vi "界面UI.vi"() -> ()   [LabVIEW 2016]
uses:
  <vilib>/Utility/config.llb/NI_LVConfig.lvlib
panel:
  in  "修改超标留样型号":bool
  out "x=y?":bool
  in  "锁":bool
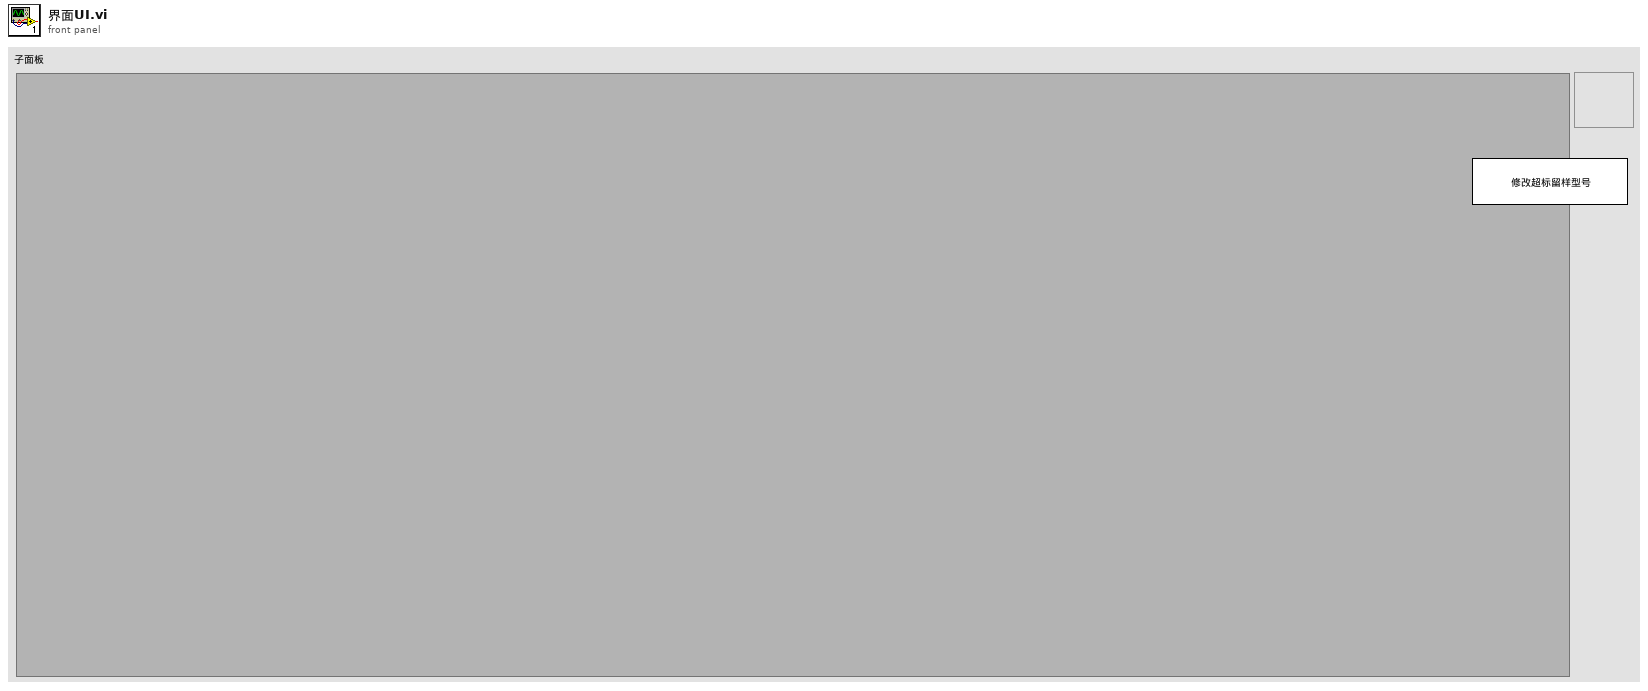
[diagram p1: front panel]
types:
  T1 = typedef "NI_LVConfig.lvlib/Config Data RefNum.ctl" = refnum<k1>
  T2 = enum16{"德润DR803M", "德润DR803L", "德润DR803F", "科盛超标留样"}
  T3 = enum32{"Bad", "Idle", "Run top level", "Running"}
  T4 = cluster{"当前瓶号：":dbl, "平行样：":dbl, "留样瓶数：":dbl, "每瓶次数：":dbl, "每次留样：":dbl, "时间间隔：":dbl, "COD联机：":u16, "氨氮联机：":u16, "4mA浓度：":dbl, "20mA浓度：":dbl, "超标浓度：":dbl, "4mA浓度：":dbl, "20mA浓度:":dbl, "超标浓度：":dbl}
  T5 = cluster{"工作状态":u16, "工作进程":u16, "仪器时间":timestamp, "采样模式":u16, "当前瓶号":dbl, "采样瓶数":dbl, "每瓶采样次数":dbl, "当前瓶已采次数":dbl, "当前瓶采样量":dbl, "采样量定量":dbl, "采样量比例":dbl, "瞬时流量":dbl, "累积流量":dbl, "外置泵状态":dbl, "采样泵状态":dbl, "采样泵方向":dbl, "采样阀":dbl, "采样瓶转盘":dbl, "排水阀":dbl, "清洗泵":dbl, "清洗管工作":dbl, "清洗管电源":dbl, "清洗管运行方向":dbl, "门状态":u16, "采水管有水检测":dbl}
  T6 = cluster{"确定":bool, "单选按钮":enum32{"德润DR803M", "德润DR803L", "德润DR803F", "科盛超标留样"}}
  T7 = enum32{"德润DR803M", "德润DR803L", "德润DR803F", "科盛超标留样"}
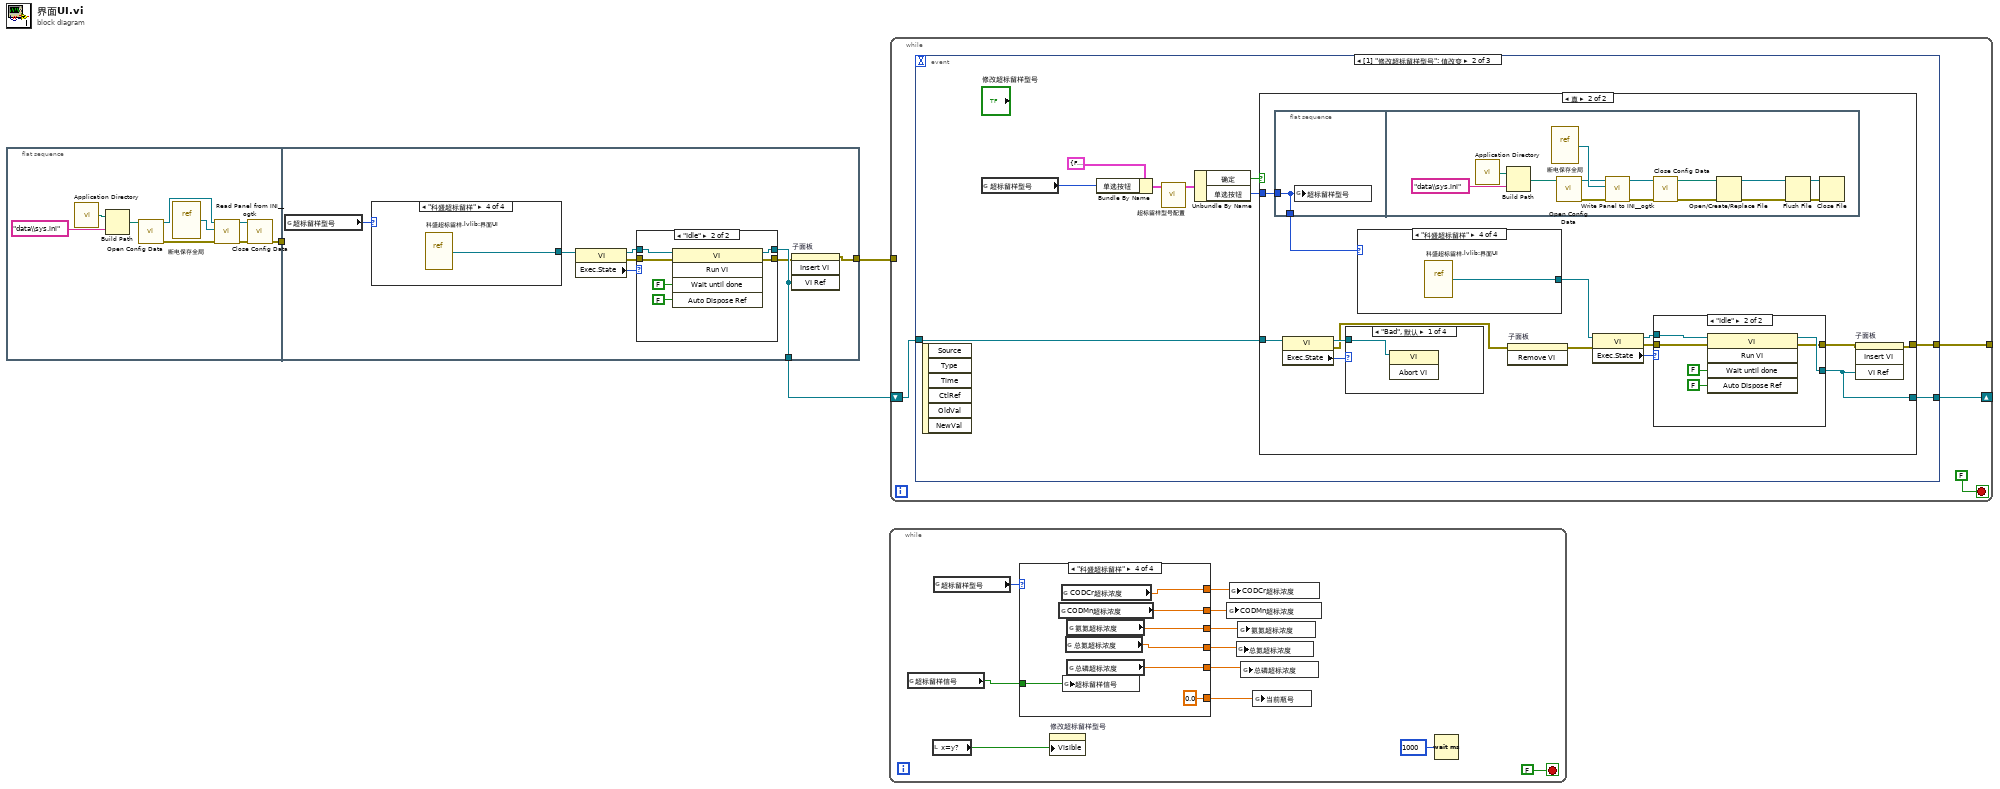
[diagram p0: block diagram]
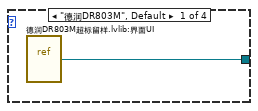
[diagram p2: hidden frame]
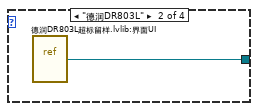
[diagram p3: hidden frame]
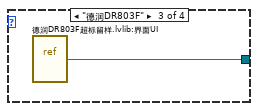
[diagram p4: hidden frame]
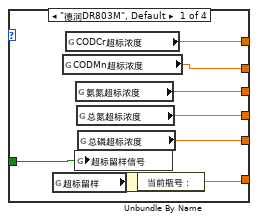
[diagram p6: hidden frame]
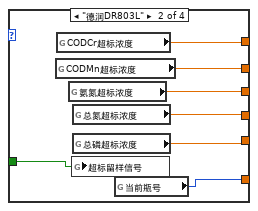
[diagram p7: hidden frame]
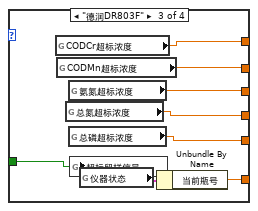
[diagram p8: hidden frame]
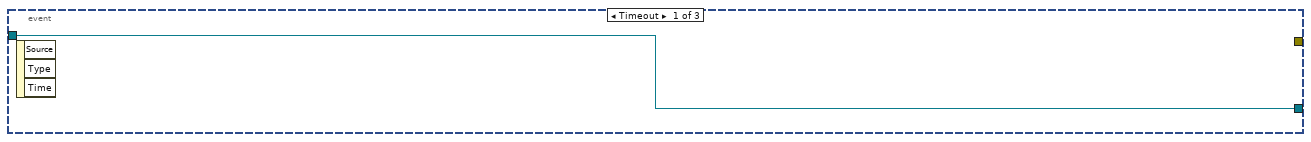
[diagram p9: hidden frame]
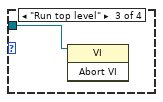
[diagram p12: hidden frame]
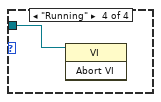
[diagram p13: hidden frame]
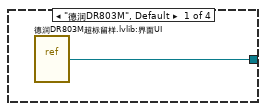
[diagram p14: hidden frame]
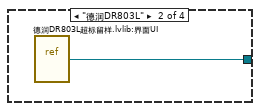
[diagram p15: hidden frame]
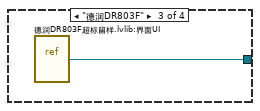
[diagram p16: hidden frame]
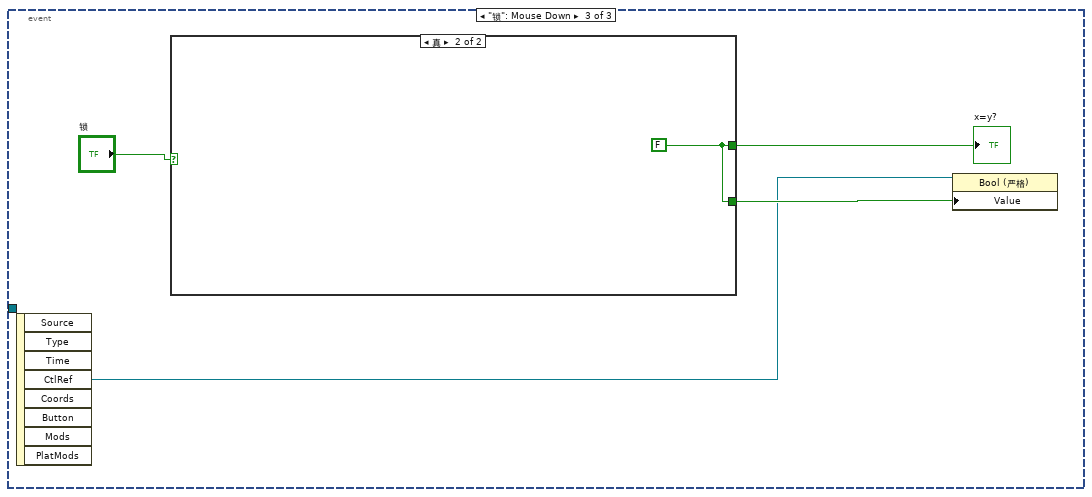
[diagram p18: hidden frame]
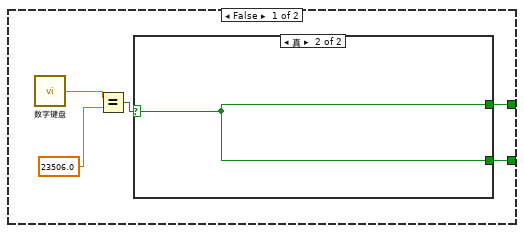
[diagram p19: hidden frame]
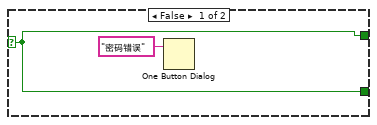
[diagram p20: hidden frame]
diagram:
  n1 = flat-sequence {
    tunnel: [w4] -> w1
    tunnel: [w15] -> w3
    tunnel: [w13] -> w2
    tunnel: w1 -> [_]
    frame #0 {
      n2 = call <vilib>:"Application Directory.vi"() -> ("Application Directory"=w5:path)
      n3 = Build Path(base path=w5, name or relative path="data\\sys.ini" ("名称或相对路径")) -> (appended path=w7:path)
      n4 = call <vilib>:"Open Config Data.vi"("configuration file path"=w7) -> ("error out"=w11:errorcluster, "refnum"=w8:T1)  [unwired: 8 in, 1 out]
      n5 = vi-ref "断电保存全局.vi"() -> (w9:refnum<vi>)
      n6 = call <userlib>:"Read Panel from INI__ogtk.vi"("error in (no error)"=w11, "VI ref"=w9, "refnum"=w8) -> ("error out"=w12:errorcluster, "refnum out"=w10:T1)  [unwired: 7 in]
      n7 = call <vilib>:"Close Config Data.vi"("error in (no error)"=w12, "refnum"=w10) -> ("error out"=w4:errorcluster)  [unwired: 8 in, 1 out]
    }
    frame #1 {
      n8 = global read "断电保存全局.vi" "超标留样型号"() -> (w16:T2)
      n9 = case shown="\"科盛超标留样\"" w16 {
        tunnel: [w21 w22 w23 w24] -> w17
        frame "德润DR803M", Default {
          n10 = vi-ref "德润DR803M超标留样.lvlib:界面UI.vi"() -> (w21:refnum<vi>)
        }
        frame "德润DR803L" {
          n11 = vi-ref "德润DR803L超标留样.lvlib:界面UI.vi"() -> (w22:refnum<vi>)
        }
        frame "德润DR803F" {
          n12 = vi-ref "德润DR803F超标留样.lvlib:界面UI.vi"() -> (w23:refnum<vi>)
        }
        frame "科盛超标留样" {
          n13 = vi-ref "科盛超标留样.lvlib:界面UI.vi"() -> (w24:refnum<vi>)
        }
      }
      n14 = property class="VI"(reference=w17) -> (reference out=w19:refnum<vi>, error out=w18:errorcluster, "Exec.State"=w20:T3)  [unwired: 1 in]
      n15 = case shown="\"Idle\"" w20 {
        tunnel: w19 -> [w26 w32]
        tunnel: [w26 w29] -> w15
        tunnel: w18 -> [w25 w28]
        tunnel: [w25 w27] -> w14
        frame "Bad", Default {
        }
        frame "Idle" {
          n16 = invoke class="VI" method="Run VI"(reference=w32, error in=w28, "Wait until done"=FALSE ("结束前等待"), "Auto Dispose Ref"=FALSE ("自动销毁引用")) -> (reference out=w29:refnum<vi>, error out=w27:errorcluster)  [unwired: 1 in, 3 out]
        }
      }
      n17 = invoke on="子面板" class="SubPnl" method="Insert VI"(error in=w14, "VI Ref"=w15) -> (error out=w13:errorcluster)  [unwired: 2 in, 3 out]
    }
  }
  n18 = while {
    stop <- FALSE stop-if-true
    n19 = global read "外部交互全局.vi" "超标留样信号"() -> (w35:bool)
    n20 = local read "x=y?"() -> (w34:bool)
    n21 = global read "断电保存全局.vi" "超标留样型号"() -> (w41:T2)
    n22 = case shown="\"科盛超标留样\"" w41 {
      tunnel: [w51 w58 w66 w73] -> w40
      tunnel: [w50 w57 w65 w72] -> w39
      tunnel: [w49 w56 w64 w71] -> w38
      tunnel: [w48 w55 w63 w70] -> w37
      tunnel: [w47 w54 w62 w69] -> w36
      tunnel: w35 -> [w46 w53 w61 w68]
      tunnel: [w44 w52 w59 0.0 ("当前瓶号")] -> w33
      frame "德润DR803M", Default {
        n23 = global read "超标留样全局.vi" "超标留样"() -> (w45:T4)
        n24 = global read "超标留样全局.vi" "CODMn超标浓度"() -> (w50:dbl)
        n25 = global read "超标留样全局.vi" "CODCr超标浓度"() -> (w51:dbl)
        n26 = global write "超标留样全局.vi" "超标留样信号"(w46) -> ()
        n27 = global read "超标留样全局.vi" "氨氮超标浓度"() -> (w49:dbl)
        n28 = global read "超标留样全局.vi" "总氮超标浓度"() -> (w48:dbl)
        n29 = global read "超标留样全局.vi" "总磷超标浓度"() -> (w47:dbl)
        n30 = Unbundle By Name(w45) -> ("当前瓶号："=w44:dbl)
      }
      frame "德润DR803L" {
        n31 = global read "串口参数断电保存全局变量.vi" "CODMn超标浓度"() -> (w57:dbl)
        n32 = global read "串口参数断电保存全局变量.vi" "CODCr超标浓度"() -> (w58:dbl)
        n33 = global read "串口参数断电保存全局变量.vi" "氨氮超标浓度"() -> (w56:dbl)
        n34 = global write "串口参数断电保存全局变量.vi" "超标留样信号"(w53) -> ()
        n35 = global read "串口参数断电保存全局变量.vi" "总氮超标浓度"() -> (w55:dbl)
        n36 = global read "串口参数断电保存全局变量.vi" "总磷超标浓度"() -> (w54:dbl)
        n37 = global read "超标留样全局.vi" "当前瓶号"() -> (w52:u16)
      }
      frame "德润DR803F" {
        n38 = global read "超标留样全局.vi" "CODCr超标浓度"() -> (w66:dbl)
        n39 = global read "超标留样全局.vi" "CODMn超标浓度"() -> (w65:dbl)
        n40 = global read "超标留样全局.vi" "总氮超标浓度"() -> (w63:dbl)
        n41 = global read "超标留样全局.vi" "氨氮超标浓度"() -> (w64:dbl)
        n42 = global read "超标留样全局.vi" "总磷超标浓度"() -> (w62:dbl)
        n43 = global write "超标留样全局.vi" "超标留样信号"(w61) -> ()
        n44 = global read "超标留样全局.vi" "仪器状态"() -> (w60:T5)
        n45 = Unbundle By Name(w60) -> ("当前瓶号"=w59:dbl)
      }
      frame "科盛超标留样" {
        n46 = global read "超标留样全局.vi" "CODMn超标浓度"() -> (w72:dbl)
        n47 = global read "超标留样全局.vi" "CODCr超标浓度"() -> (w73:dbl)
        n48 = global write "超标留样全局.vi" "超标留样信号"(w68) -> ()
        n49 = global read "超标留样全局.vi" "总氮超标浓度"() -> (w70:dbl)
        n50 = global read "超标留样全局.vi" "氨氮超标浓度"() -> (w71:dbl)
        n51 = global read "超标留样全局.vi" "总磷超标浓度"() -> (w69:dbl)
      }
    }
    n52 = property on="修改超标留样型号" class="Bool"("Visible"=w34) -> ()  [unwired: 2 in, 2 out]
    n53 = global write "外部交互全局.vi" "CODMn超标浓度"(w39) -> ()
    n54 = global write "外部交互全局.vi" "CODCr超标浓度"(w40) -> ()
    n55 = global write "外部交互全局.vi" "总氮超标浓度"(w37) -> ()
    n56 = global write "外部交互全局.vi" "氨氮超标浓度"(w38) -> ()
    n57 = global write "外部交互全局.vi" "总磷超标浓度"(w36) -> ()
    n58 = global write "外部交互全局.vi" "当前瓶号"(w33) -> ()
    n59 = Wait (ms)(milliseconds to wait=u32 1000 ("等待时间（毫秒）")) -> ()  [unwired: 1 out]
  }
  n60 = while {
    tunnel: [w77] -> _
    tunnel: w2 -> [_]
    shift-right: [w75] -> _
    shift-left: w3 -> [w74]
    stop <- FALSE stop-if-true
    n61 = event shown="[1] \"修改超标留样型号\": 值改变" {
      selector: _ -> [_ _ _]
      dyn-events: _ -> [_ _ _]
      timeout: _ -> [_ _ _]
      tunnel: [_ w81 _] -> w77
      tunnel: [w78 w80 _] -> w75
      tunnel: w74 -> [w78 w79 _]
      event Timeout {
        n62 = event-data() -> ()  [unwired: 1 in, 3 out]
      }
      event "修改超标留样型号": Value Change {
        n63 = event-data() -> ()  [unwired: 1 in, 6 out]
        n64 = global read "断电保存全局.vi" "超标留样型号"() -> (w87:T2)
        n65 = Bundle By Name(cluster=T6 {"确定"=FALSE, "单选按钮"=enum."德润DR803F"} ("输入"), "单选按钮"=w87) -> (w85:T6)
        n66 = call "超标留样型号配置.vi"("输入"=w85) -> ("输出"=w84:T6)  [unwired: 10 in]
        n67 = Unbundle By Name(w84) -> ("确定"=w82:bool, "单选按钮"=w83:T7)
        n68 = case shown="真" w82 {
          tunnel: w83 -> [_ w102]
          tunnel: [_ w91] -> w81
          tunnel: [w88 w92] -> w80
          tunnel: w79 -> [w88 w96]
          frame False {
          }
          frame True {
            n69 = flat-sequence {
              tunnel: w102 -> [w118]
              tunnel: [w118] -> w97
              frame #0 {
                n70 = global write "断电保存全局.vi" "超标留样型号"(w118) -> ()
              }
              frame #1 {
                n71 = call <vilib>:"Application Directory.vi"() -> ("Application Directory"=w120:path)
                n72 = Build Path(base path=w120, name or relative path="data\\sys.ini" ("名称或相对路径")) -> (appended path=w121:path)
                n73 = vi-ref "断电保存全局.vi"() -> (w123:refnum<vi>)
                n74 = call <vilib>:"Open Config Data.vi"("configuration file path"=w121) -> ("error out"=w125:errorcluster, "refnum"=w122:T1)  [unwired: 8 in, 1 out]
                n75 = call <userlib>:"Write Panel to INI__ogtk.vi"("error in (no error)"=w125, "VI ref"=w123, "refnum"=w122) -> ("error out"=w126:errorcluster, "refnum out"=w124:T1)  [unwired: 7 in]
                n76 = call <vilib>:"Close Config Data.vi"("error in (no error)"=w126, "refnum"=w124) -> ("error out"=w131:errorcluster, "file path"=w132:path)  [unwired: 8 in]
                n77 = Open/Create/Replace File(file path (use dialog)=w132, error in=w131) -> (refnum out=w128:refnum<file>, error out=w127:errorcluster)  [unwired: 4 in, 1 out]
                n78 = Flush File(refnum=w128, error in=w127) -> (refnum out=w129:refnum<file>, error out=w130:errorcluster)
                n79 = Close File(refnum=w129, error in=w130) -> ()  [unwired: 2 out]
              }
            }
            n80 = property class="VI"(reference=w96) -> (reference out=w94:refnum<vi>, error out=w90:errorcluster, "Exec.State"=w95:T3)  [unwired: 1 in]
            n81 = case shown="\"Bad\", 默认" w95 {
              tunnel: w94 -> [w103 _ w104 w105]
              frame "Bad", Default {
                n82 = invoke class="VI" method="Abort VI"(reference=w103) -> ()  [unwired: 2 in, 3 out]
              }
              frame "Idle" {
              }
              frame "Run top level" {
                n83 = invoke class="VI" method="Abort VI"(reference=w104) -> ()  [unwired: 2 in, 3 out]
              }
              frame "Running" {
                n84 = invoke class="VI" method="Abort VI"(reference=w105) -> ()  [unwired: 2 in, 3 out]
              }
            }
            n85 = case shown="\"科盛超标留样\"" w97 {
              tunnel: [w106 w107 w108 w109] -> w98
              frame "德润DR803M", Default {
                n86 = vi-ref "德润DR803M超标留样.lvlib:界面UI.vi"() -> (w106:refnum<vi>)
              }
              frame "德润DR803L" {
                n87 = vi-ref "德润DR803L超标留样.lvlib:界面UI.vi"() -> (w107:refnum<vi>)
              }
              frame "德润DR803F" {
                n88 = vi-ref "德润DR803F超标留样.lvlib:界面UI.vi"() -> (w108:refnum<vi>)
              }
              frame "科盛超标留样" {
                n89 = vi-ref "科盛超标留样.lvlib:界面UI.vi"() -> (w109:refnum<vi>)
              }
            }
            n90 = invoke on="子面板" class="SubPnl" method="Remove VI"(error in=w90) -> (error out=w89:errorcluster)  [unwired: 2 in, 2 out]
            n91 = property class="VI"(reference=w98, error in=w89) -> (reference out=w100:refnum<vi>, error out=w99:errorcluster, "Exec.State"=w101:T3)
            n92 = case shown="\"Idle\"" w101 {
              tunnel: w100 -> [w111 w117]
              tunnel: [w111 w114] -> w92
              tunnel: w99 -> [w110 w113]
              tunnel: [w110 w112] -> w93
              frame "Bad", Default {
              }
              frame "Idle" {
                n93 = invoke class="VI" method="Run VI"(reference=w117, error in=w113, "Wait until done"=FALSE ("结束前等待"), "Auto Dispose Ref"=FALSE ("自动销毁引用")) -> (reference out=w114:refnum<vi>, error out=w112:errorcluster)  [unwired: 1 in, 3 out]
              }
            }
            n94 = invoke on="子面板" class="SubPnl" method="Insert VI"(error in=w93, "VI Ref"=w92) -> (error out=w91:errorcluster)  [unwired: 2 in, 3 out]
          }
        }
      }
      event "锁": Mouse Down {
        n95 = event-data() -> ("CtlRef"=w134:refnum<vi>)  [unwired: 1 in, 7 out]
        n96 = case shown="真" "锁" {
          tunnel: [w138 w145] -> w136
          tunnel: [w137 w145] -> w135
          frame False {
            n97 = call "数字键盘.vi"() -> ("NewNumber"=w141:sgl)  [unwired: 1 in]
            n98 = Equal?(x=w141, y=sgl 23506.0) -> (x = y?=w139:bool)
            n99 = case shown="真" w139 {
              selector: w139 -> [w142 w144]
              tunnel: [w142 w144] -> w138
              tunnel: [w142 w144] -> w137
              frame False {
                n100 = One Button Dialog(message="密码错误" ("消息")) -> ()  [unwired: 1 in, 1 out]
              }
              frame True {
              }
            }
          }
          frame True {
            w145 = FALSE
          }
        }
        "x=y?" <- w136
        n101 = property class="Bool (严格)"(reference=w134, "Value"=w135) -> ()  [unwired: 1 in, 2 out]
      }
    }
  }
